vi "例7-6（2).vi"() -> ()   [LabVIEW 2019]
panel:
  out "波形图表":dbl[](graph)
  in  "停止":bool
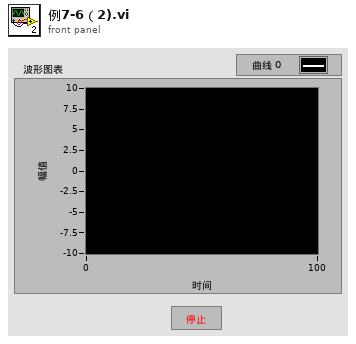
[diagram p1: front panel]
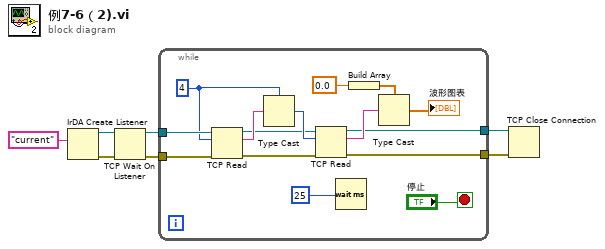
[diagram p0: block diagram]
diagram:
  n1 = IrDA Create Listener(10:"current" ("服务名称")) -> (0:w7:errorcluster, 3:w6:refnum<k19>)  [unwired: 1 in]
  n2 = TCP Wait On Listener(8:w7, 11:w6) -> (0:w3:errorcluster, 3:w4:refnum<k19>)  [unwired: 2 in, 3 out]
  n3 = while {
    tunnel: w4 -> [w22]
    tunnel: w3 -> [w21]
    tunnel: [w11] -> w2
    tunnel: [w10] -> w1
    stop <- "停止" stop-if-true
    w18 = 4
    n4 = TCP Read(connection ID=w22, bytes to read=w18, error in (no error)=w21) -> (connection ID out=w17:refnum<k19>, data out=w20:string, error out=w16:errorcluster)  [unwired: 2 in]
    n5 = Type Cast(type=w18, x=w20) -> (*(type *) &x=w19:i32)
    n6 = TCP Read(connection ID=w17, bytes to read=w19, error in (no error)=w16) -> (connection ID out=w11:refnum<k19>, data out=w15:string, error out=w10:errorcluster)  [unwired: 2 in]
    n7 = Wait (ms)(milliseconds to wait=25) -> ()  [unwired: 1 out]
    n8 = Build Array(0.0) -> (w12:dbl[])
    n9 = Type Cast(type=w12, x=w15) -> (*(type *) &x=→"波形图表":dbl[])
  }
  n10 = TCP Close Connection(connection ID=w2, error in (no error)=w1) -> ()  [unwired: 1 in, 2 out]
